vi "SQL_Sandbox.vi"() -> ()   [LabVIEW 2017]
uses:
  <vilib>/addons/database/NI_Database_API.lvlib
  <vilib>/addons/database/Connection.llb/DB Tools Open Connec (String).vi
  <vilib>/addons/database/Connection.llb/Conn Execute.vi
  <vilib>/addons/database/Recordset.llb/Rec Fetch Recordset Data (R).vi
  <vilib>/addons/database/_DB Variant To Data/Database Variant To Data.xnode
panel:
  out "error out":errorcluster
  in  "data":variant[][](array[variant])
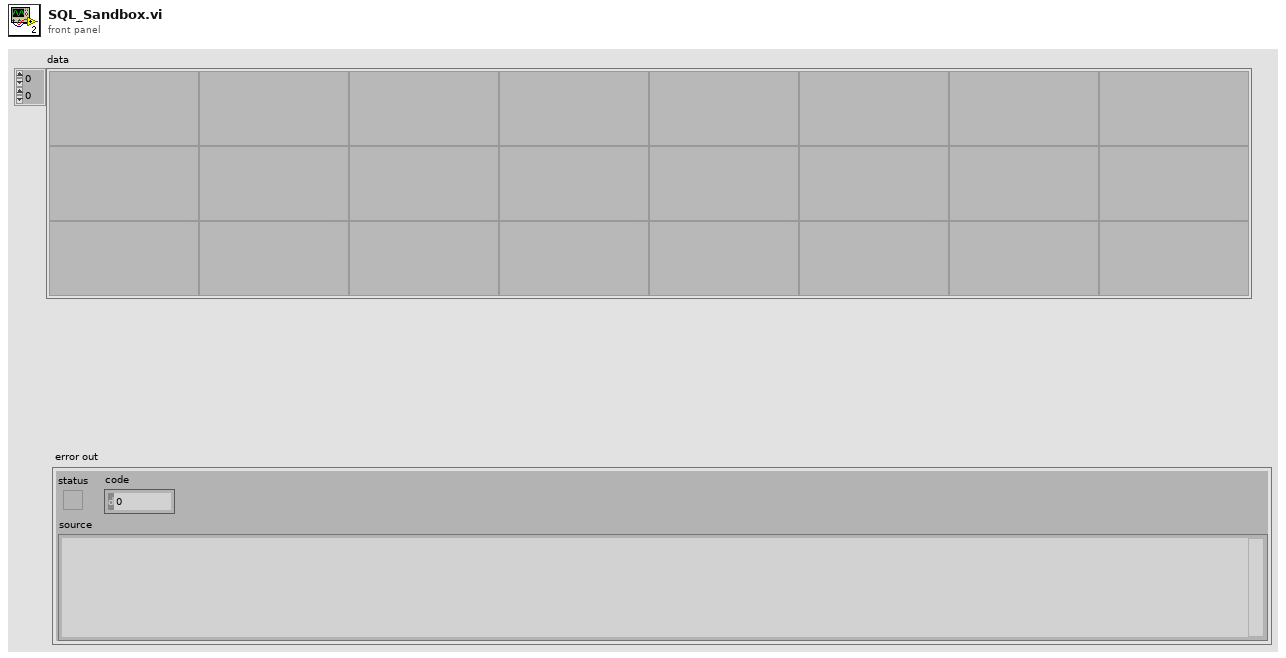
[diagram p1: front panel]
types:
  T1 = typedef "NI_Database_API.lvlib/Conn ObjectReference.ctl" = refnum<k1>
  T2 = typedef "NI_Database_API.lvlib/Rec ObjectReference.ctl" = refnum<k1>
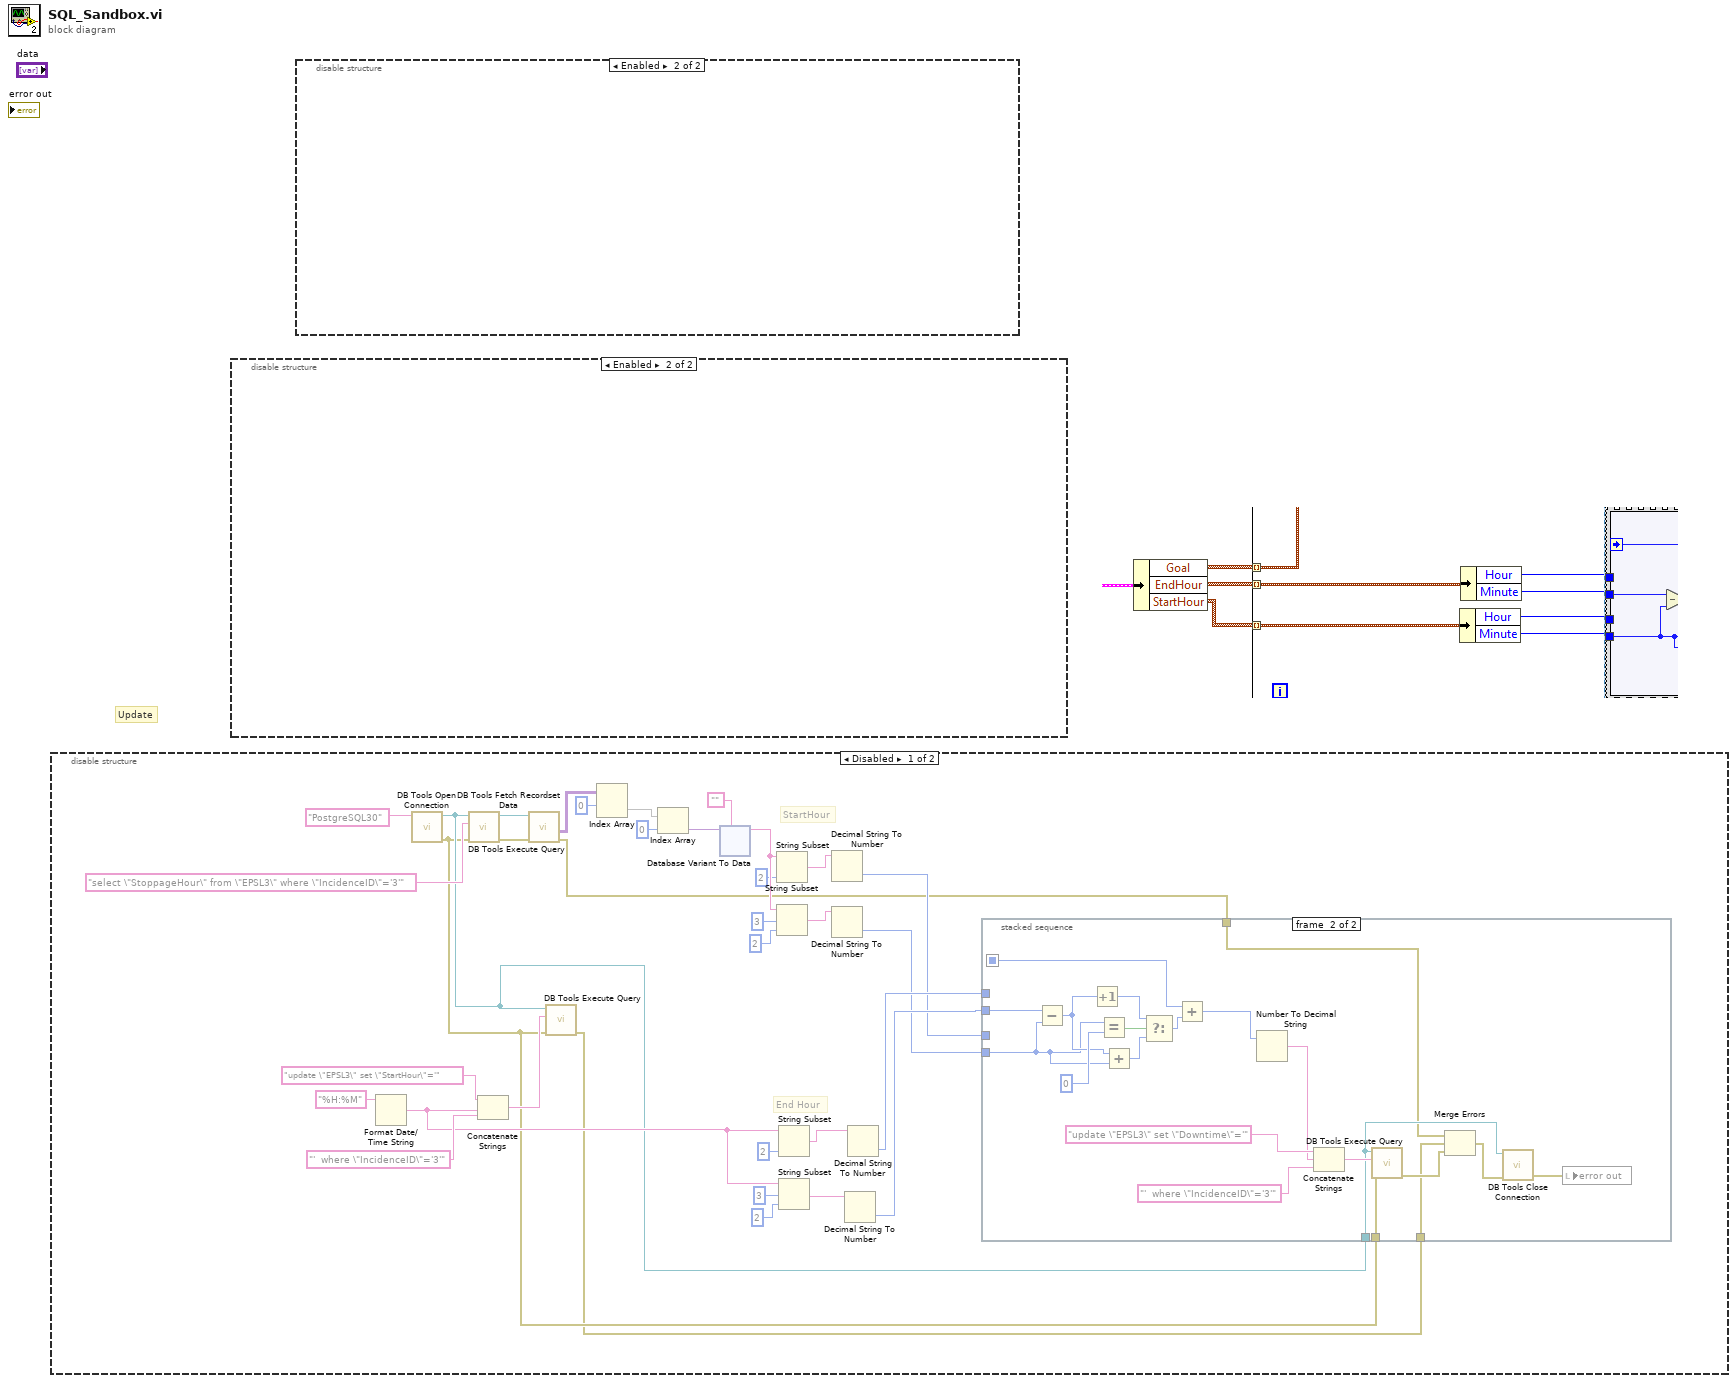
[diagram p0: block diagram]
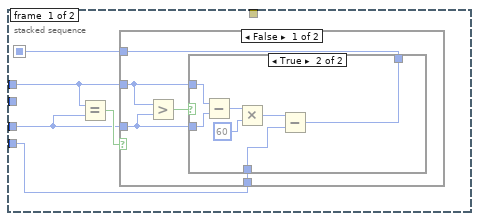
[diagram p2: hidden frame]
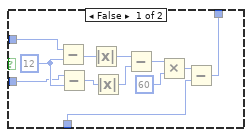
[diagram p3: hidden frame]
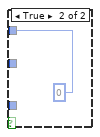
[diagram p4: hidden frame]
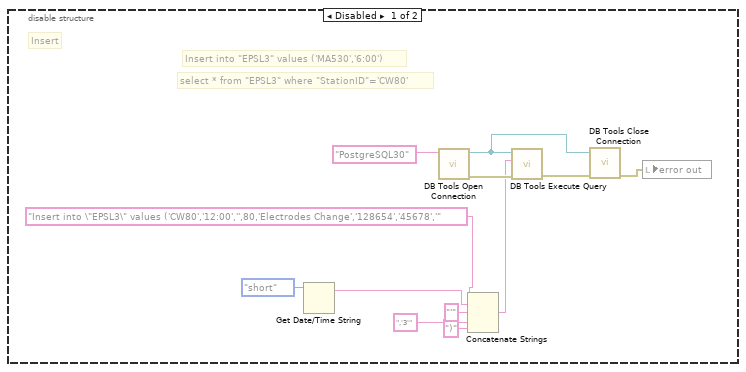
[diagram p6: hidden frame]
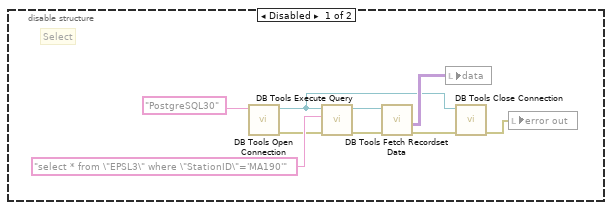
[diagram p7: hidden frame]
diagram:
  # "Update"
  n1 = disable-structure shown="Disabled" {
    frame Disabled {
      # "End Hour"
      # "StartHour"
      n2 = Format Date/Time String(time format string (%c)="%H:%M") -> (date/time string=w13:string)  [unwired: 2 in]
      n3 = call-poly <vilib>:"DB Tools Open Connection.vi"("connection information"="PostgreSQL30") -> ("error out"=w3:errorcluster, "connection reference"=w4:T1)  [unwired: 7 in]
      n4 = call-poly <vilib>:"DB Tools Execute Query.vi"("error in (no error)"=w3, "SQL query"="select \"StoppageHour\" from \"EPSL3\" where \"IncidenceID\"='3'", "connection reference"=w4) -> ("error out"=w33:errorcluster, "recordset reference"=w32:T2)  [unwired: 5 in]
      n5 = Concatenate Strings("update \"EPSL3\" set \"StartHour\"='" ("SQL query"), w13, "'  where \"IncidenceID\"='3'") -> (w18:string)
      n6 = call-poly <vilib>:"DB Tools Fetch Recordset Data.vi"("error in (no error)"=w33, "recordset reference"=w32) -> ("error out"=w1:errorcluster, "recordset data"=w27:variant[][])  [unwired: 3 in, 1 out]
      n7 = call-poly <vilib>:"DB Tools Execute Query.vi"("error in (no error)"=w3, "SQL query"=w18, "connection reference"=w4) -> ("error out"=w2:errorcluster)  [unwired: 5 in, 1 out]
      n8 = Index Array(array=w27, index (row)=0) -> (element=w29:variant[])  [unwired: 1 in]
      n9 = Index Array(array=w29, index=0) -> (element=w26:variant)
      n10 = xnode "Database Variant To Data"("database variant"=w26, "type"="") -> ("data"=w24:string)  [unwired: 1 in, 1 out]
      n11 = String Subset(string=w24, length (rest)=2 ("length (rest)")) -> (substring=w8:string)  [unwired: 1 in]
      n12 = String Subset(string=w24, offset (0)=3 ("length (rest)"), length (rest)=2 ("length (rest)")) -> (substring=w7:string)
      n13 = String Subset(string=w13, length (rest)=2 ("length (rest)")) -> (substring=w12:string)  [unwired: 1 in]
      n14 = String Subset(string=w13, offset (0)=3 ("length (rest)"), length (rest)=2 ("length (rest)")) -> (substring=w10:string)
      n15 = Decimal String To Number(string=w8) -> (number=w6:i32)  [unwired: 2 in, 1 out]
      n16 = Decimal String To Number(string=w7) -> (number=w5:i32)  [unwired: 2 in, 1 out]
      n17 = Decimal String To Number(string=w10) -> (number=w9:i32)  [unwired: 2 in, 1 out]
      n18 = Decimal String To Number(string=w12) -> (number=w11:i32)  [unwired: 2 in, 1 out]
      n19 = stacked-sequence {
        seq-local: [w38 _] -> [_ w80]
        tunnel: w9 -> [_ w85]
        tunnel: w5 -> [w35 w78]
        tunnel: w11 -> [w37 _]
        tunnel: w6 -> [w36 _]
        tunnel: w4 -> [_ w71]
        tunnel: w3 -> [_ w72]
        tunnel: w2 -> [_ w69]
        tunnel: w1 -> [_ w68]
        frame #0 {
          n20 = Equal?(x=w37, y=w36) -> (x = y?=w39:bool)
          n21 = case shown="False" w39 {
            tunnel: [w43 0] -> w38
            tunnel: w37 -> [w42 _]
            tunnel: w36 -> [w41 _]
            tunnel: w35 -> [w44 _]
            frame False {
              n22 = Greater?(x=w42, y=w41) -> (0:w40:bool)
              n23 = case shown="True" w40 {
                tunnel: w42 -> [w52 w63]
                tunnel: w41 -> [w49 w62]
                tunnel: w44 -> [w51 w58]
                tunnel: [w53 w57] -> w43
                frame False {
                  w50 = 12
                  n24 = Subtract(x=w52, y=w50) -> (x-y=w47:i32)
                  n25 = Subtract(x=w49, y=w50) -> (x-y=w46:i32)
                  n26 = Absolute Value(x=w47) -> (abs(x)=w48:i32)
                  n27 = Absolute Value(x=w46) -> (abs(x)=w45:i32)
                  n28 = Subtract(x=w48, y=w45) -> (x-y=w55:i32)
                  n29 = Multiply(x=w55, y=60) -> (x*y=w56:i32)
                  n30 = Subtract(x=w56, y=w51) -> (x-y=w53:i32)
                }
                frame True {
                  n31 = Subtract(x=w63, y=w62) -> (x-y=w61:i32)
                  n32 = Multiply(x=w61, y=60) -> (x*y=w59:i32)
                  n33 = Subtract(x=w59, y=w58) -> (x-y=w57:i32)
                }
              }
            }
            frame True {
            }
          }
        }
        frame #1 {
          n34 = Subtract(x=w85, y=w78) -> (x-y=w79:i32)
          n35 = Increment(x=w79) -> (x+1=w82:i32)
          n36 = Equal?(x=w78, y=0) -> (x = y?=w83:bool)
          n37 = Add(x=w79, y=w78) -> (x+y=w77:i32)
          n38 = Select(t=w82, s=w83, f=w77) -> (s? t:f=w81:i32)
          n39 = Add(x=w80, y=w81) -> (x+y=w65:i32)
          n40 = Number To Decimal String(number=w65) -> (decimal integer string=w75:string)  [unwired: 1 in]
          n41 = Concatenate Strings("update \"EPSL3\" set \"Downtime\"='" ("SQL query"), w75, "'  where \"IncidenceID\"='3'") -> (w73:string)
          n42 = call-poly <vilib>:"DB Tools Execute Query.vi"("error in (no error)"=w72, "SQL query"=w73, "connection reference"=w71) -> ("error out"=w70:errorcluster)  [unwired: 5 in, 1 out]
          n43 = Merge Errors(w68, w69, w70) -> (w67:errorcluster)
          n44 = call <vilib>:"DB Tools Close Connection.vi"("error in (no error)"=w67, "connection reference"=w71) -> ("error out"=w66:errorcluster)  [unwired: 5 in]
          n45 = local write "error out"(w66) -> ()
        }
      }
    }
    frame Enabled {
    }
  }
  n46 = disable-structure shown="Enabled" {
    frame Disabled {
      # "Insert"
      # "select * from \"EPSL3\" where \"StationID\"='CW80'"
      # "Insert into \"EPSL3\" values ('MA530','6:00')"
      n47 = Get Date/Time String(date format (0)=enum16{"short", "long", "abbreviated"}."short") -> (date string=w120:string)  [unwired: 2 in, 1 out]
      n48 = call-poly <vilib>:"DB Tools Open Connection.vi"("connection information"="PostgreSQL30") -> ("error out"=w127:errorcluster, "connection reference"=w125:T1)  [unwired: 7 in]
      n49 = Concatenate Strings("Insert into \"EPSL3\" values ('CW80','12:00','',80,'Electrodes Change','128654','45678','" ("SQL query"), w120, "'" ("string"), ",'3'" ("string"), ")" ("string")) -> (w123:string)
      n50 = call-poly <vilib>:"DB Tools Execute Query.vi"("error in (no error)"=w127, "SQL query"=w123, "connection reference"=w125) -> ("error out"=w126:errorcluster)  [unwired: 5 in, 1 out]
      n51 = call <vilib>:"DB Tools Close Connection.vi"("error in (no error)"=w126, "connection reference"=w125) -> ("error out"=w128:errorcluster)  [unwired: 5 in]
      n52 = local write "error out"(w128) -> ()
    }
    frame Enabled {
    }
  }
  n53 = disable-structure shown="Enabled" {
    frame Disabled {
      # "Select"
      n54 = call-poly <vilib>:"DB Tools Open Connection.vi"("connection information"="PostgreSQL30") -> ("error out"=w137:errorcluster, "connection reference"=w130:T1)  [unwired: 7 in]
      n55 = call-poly <vilib>:"DB Tools Execute Query.vi"("error in (no error)"=w137, "SQL query"="select * from \"EPSL3\" where \"StationID\"='MA190'", "connection reference"=w130) -> ("error out"=w133:errorcluster, "recordset reference"=w134:T2)  [unwired: 5 in]
      n56 = call-poly <vilib>:"DB Tools Fetch Recordset Data.vi"("error in (no error)"=w133, "recordset reference"=w134) -> ("error out"=w132:errorcluster, "recordset data"=w131:variant[][])  [unwired: 3 in, 1 out]
      n57 = local write "data"(w131) -> ()
      n58 = call <vilib>:"DB Tools Close Connection.vi"("error in (no error)"=w132, "connection reference"=w130) -> ("error out"=w136:errorcluster)  [unwired: 5 in]
      n59 = local write "error out"(w136) -> ()
    }
    frame Enabled {
    }
  }
